vi "project review2.vi"() -> ()   [LabVIEW 2019]
uses:
  <vilib>/Instr/_visa.llb/VISA Configure Serial Port (Instr).vi
panel:
  out "Hopper 2":dbl(slide) scale=0.0..100.0
  out "Hopper":dbl(slide) scale=0.0..100.0
  out "Meter 2":dbl(knob) scale=0.0..10.0
  out "Meter":dbl(knob) scale=0.0..10.0
  out "Boolean array":bool[](array[boolean])
  out "element":u8
  in  "milliseconds":u32
  out "String":string
  out "Numeric":u8
  in  "Array":bool[](array[boolean])
  in  "Motor Speed":u8(slide) scale=0.0..10.0
  in  "flow control":u16(ring) items=["None", "XON/XOFF", "RTS/CTS", "XON/XOFF & RTS/CTS", "DTR/DSR", "XON/XOFF & DTR/DSR"]
  in  "stop bits":u16(ring)=10 items=["1.0"=10, "1.5"=15, "2.0"=20]
  in  "parity":enum16{"None", "Odd", "Even", "Mark", "Space"}(ring)
  in  "data bits (8)":u16=8 min=5 max=8 step=1
  in  "baud rate (9600)":u32=9600
  in  "VISA resource name":refnum<visa-resource-name>
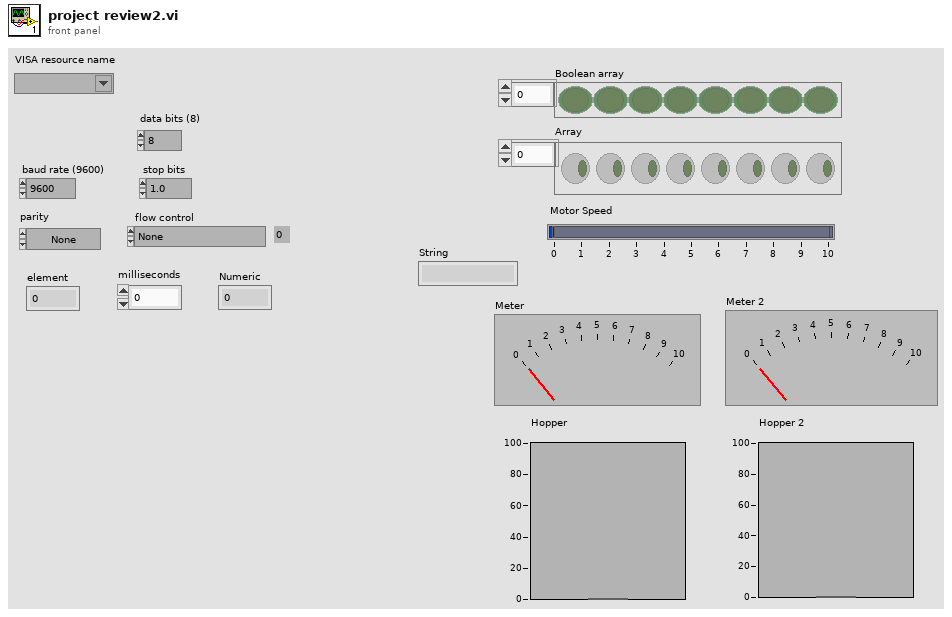
[diagram p1: front panel]
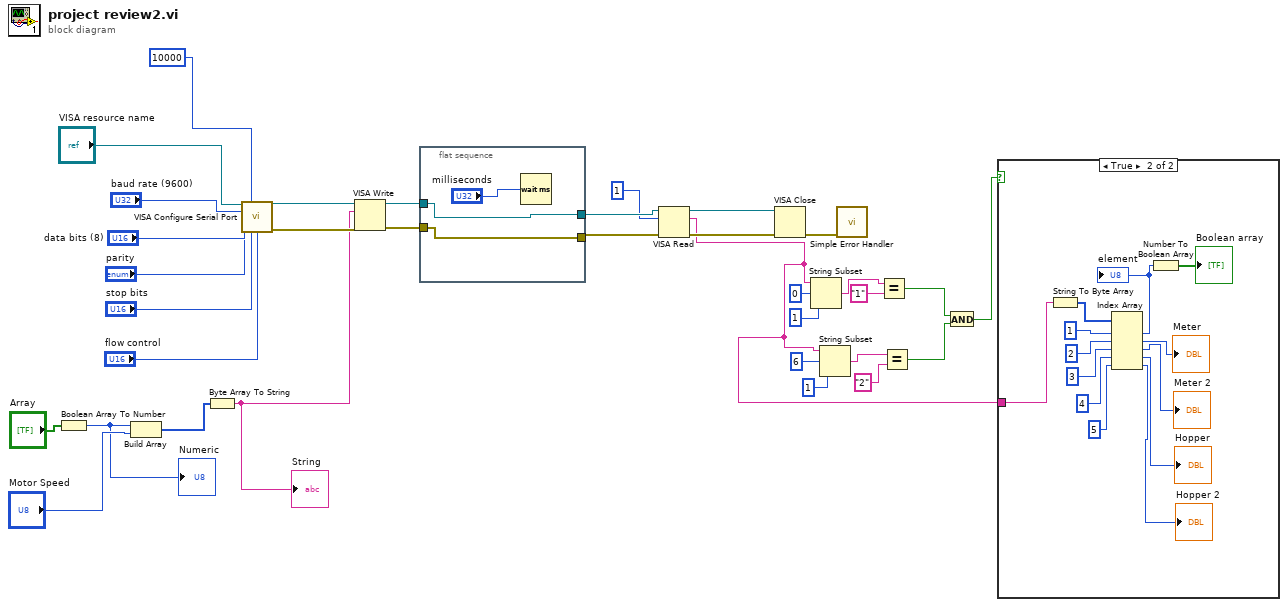
[diagram p0: block diagram]
diagram:
  n1 = Boolean Array To Number(Boolean array="Array") -> (number=w26:u32)
  "Numeric" <- w26
  n2 = Build Array(w26, "Motor Speed") -> (w25:u32[])
  n3 = Byte Array To String(unsigned byte array=w25) -> (string=w22:string)
  "String" <- w22
  n4 = call-poly "VISA Configure Serial Port"("VISA resource name"="VISA resource name", "timeout (10sec)"=u32 10000, "baud rate (9600)"="baud rate (9600)", "data bits (8)"="data bits (8)", "parity (0:none)"="parity", "stop bits (10: 1 bit)"="stop bits", "flow control (0:none)"="flow control") -> ("VISA resource name out"=w24:refnum<visa-resource-name>, "error out"=w23:errorcluster)  [unwired: 7 in]
  n5 = VISA Write(VISA resource name=w24, write buffer=w22, error in (no error)=w23) -> (VISA resource name out=w20:refnum<visa-resource-name>, error out=w21:errorcluster)  [unwired: 1 out]
  n6 = flat-sequence {
    tunnel: w21 -> [w36]
    tunnel: w20 -> [w37]
    tunnel: [w37] -> w19
    tunnel: [w36] -> w18
    frame #0 {
      n7 = Wait (ms)(milliseconds to wait="milliseconds") -> ()  [unwired: 1 out]
    }
  }
  n8 = VISA Read(VISA resource name=w19, byte count=u32 1, error in (no error)=w18) -> (VISA resource name out=w17:refnum<visa-resource-name>, read buffer=w3:string, error out=w16:errorcluster)  [unwired: 1 out]
  n9 = VISA Close(VISA resource name=w17, error in (no error)=w16) -> (error out=w1:errorcluster)
  n10 = String Subset(string=w3, offset (0)=0, length (rest)=1 ("length (rest)")) -> (substring=w10:string)
  n11 = String Subset(string=w3, offset (0)=6, length (rest)=1 ("length (rest)")) -> (substring=w8:string)
  n12 = call <vilib>:"Simple Error Handler.vi"("error in (no error)"=w1) -> ()  [unwired: 4 in, 5 out]
  n13 = Equal?(x=w10, y="1") -> (x = y?=w6:bool)
  n14 = Equal?(x=w8, y="2") -> (x = y?=w5:bool)
  n15 = And(x=w6, y=w5) -> (x .and. y?=w4:bool)
  n16 = case shown="True" w4 {
    tunnel: w3 -> [_ w50]
    frame False {
    }
    frame True {
      n17 = String To Byte Array(string=w50) -> (unsigned byte array=w44:u8[])
      n18 = Index Array(array=w44, index #1=1 ("index"), index #2=2 ("index"), index #3=3 ("index"), index #4=4 ("index"), index #5=5 ("index")) -> (element #1=w43:u8, element #2=→"Meter":u8, element #3=→"Meter 2":u8, element #4=→"Hopper":u8, element #5=→"Hopper 2":u8)
      "element" <- w43
      n19 = Number To Boolean Array(number=w43) -> (Boolean array=→"Boolean array":bool[])
    }
  }
